vi "GetSpeed.vi"(8 "error in (no error)":errorcluster, 11 "StepMotor in":refnum<class "StepMotor.lvclass">) -> (0 "error out":errorcluster, 2 "Скорость":dbl, 3 "StepMotor out":refnum<class "StepMotor.lvclass">)   [LabVIEW 2010, in "StepMotor.lvclass"]
uses:
  StepMotor.lvclass
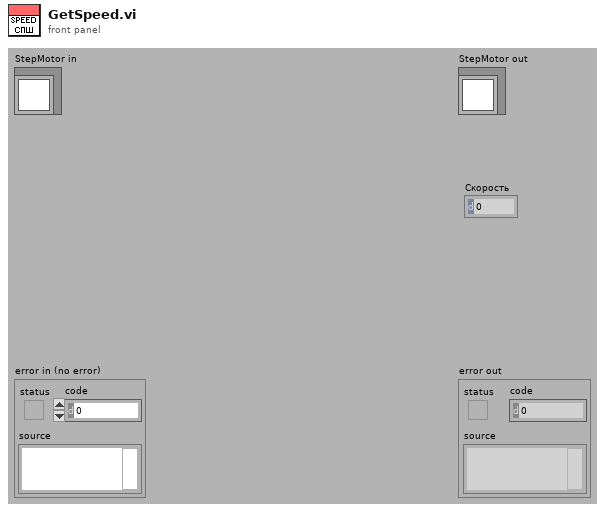
[diagram p1: front panel]
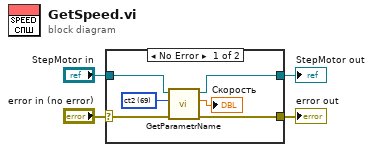
[diagram p0: block diagram]
diagram:
  n1 = case shown="No Error" "error in (no error)" {
    selector: "error in (no error)" -> [w8 w12]
    tunnel: [w5 w12] -> w3
    tunnel: [w6 w11] -> w1
    tunnel: "StepMotor in" -> [w7 w11]
    frame No Error {
      w9 = 69 items=["cp1", "cp2", "cp3", "cp4", "cp5", "cp6", "cp7", "cp8", "cp9", "cp10", "cp11", "cp12", "vp1", "vp2", "vp16", "vp3", "vp4", "vp5", "vp6", "vp7", "vp8", "vp9", "vp10", "vp11", "vp12", "vp13", "vp14", "vp15", "vp17", "vp18", "vp19", "vp20", "vp21", "vp22", "vp23", "vp24", "vp25", "vp26", "pp1", "pp2", "pp3", "pp5", "pp6", "pp7", "pp8", "pp9", "pp10", "pp11", "ss1", "ss2", "ss3", "ss4", "ss5", "ss6", "ss7", "ss8", "ss9", "ss10", "ss11", "ss12", "ss13", "ss14", "ss15", "si1", "si2", "ss16", "ss17", "ss18", "ct1", "ct2", "ct3", "dd1", "dd6", "dd3", "dd9", "dd2", "dd4", "dd5", "dd21", "dd7", "dd8", "dd20", "dd10", "dd19", "dd12", "dd11", "dd13", "dd14", "dd15", "dd16", "dd17", "dd18", "dd22", "dd23", "dd24", "dd25", "dd26", "dd27", "dd28", "dd29", "dd30", "dd31", "dd32", "dd33", "dd34", "st1", "st2", "st3", "st4", "st5", "st6", "st7", "st8", "st9", "st10", "st11", "st12", "st13", "st14", "tp1", "tp3", "tp2", "tp5", "tp6", "ip0", "ip1", "ip2", "ip3", "ip4", "ip5", "ip6", "ip7", "ip8", "ip9", "ip10", "ip11", "ip12", "ip13", "ip14", "ip15", "ip16", "ip17", "ip18", "ip19", "ip20", "ep1", "ep2", "ep3", "ep4", "ep5", "ep6", "ep7", "up0", "up1", "up2", "up3", "up4", "up5", "up6", "up7", "up8", "up9", "up10", "up11", "up12", "up13", "up14", "up15", "up16", "up17", "up18", "up19", "up20", "up21", "up22", "up23", "up24", "io0", "io1", "io2", "io3", "io4", "io5", "io6", "io7", "io8", "io9", "io10", "io11", "io12", "io13", "io14", "pd1", "pd2", "pd3", "pd4", "pd5", "pd6", "pd7", "pd8", "pd9", "pd10", "pd11", "pd12", "pd13", "pd14", "pd15", "pd16", "pd17", "pd18", "pd19"] ("Имя параметра")
      n2 = call "GetParametrName.vi"("error in (no error)"=w8, "Имя параметра"=w9, "StepMotor in"=w7) -> ("error out"=w5:errorcluster, "Значение"=→"Скорость":dbl, "StepMotor out"=w6:refnum<class "StepMotor.lvclass">)  [unwired: 6 in]
    }
    frame Error {
    }
  }
  "error out" <- w3
  "StepMotor out" <- w1
